vi "Create and Format PNG Image Link.vi"(8 "Error In":errorcluster, 11 "Image Name Cluster":T1) -> (0 "Error Out":errorcluster, 3 "Image Link":string)   [LabVIEW 2017]
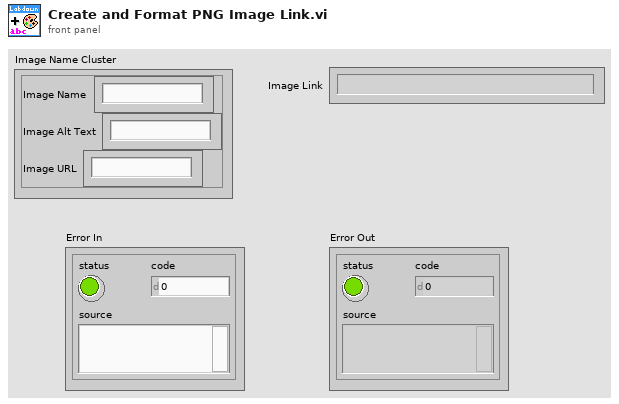
[diagram p1: front panel]
types:
  T1 = cluster{"Image Name":string, "Image Alt Text":string, "Image URL":string}
  T2 = enum16{"Header 1", "Header 2", "Header 3", "Header 4", "Header 5", "Header 6"}
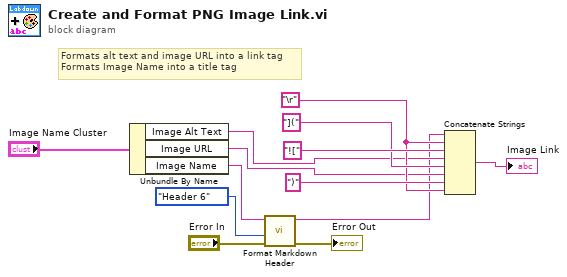
[diagram p0: block diagram]
diagram:
  w8 = "\r"
  # "Formats alt text and image URL into a link tag\nFormats Image Name into a title tag"
  n1 = Unbundle By Name("Image Name Cluster") -> ("Image Alt Text"=w4:string, "Image URL"=w2:string, "Image Name"=w3:string)
  n2 = call "Format Markdown Header.vi"("Error In"="Error In", "Header Size"=T2."Header 6", "Unformatted Heading Input"=w3) -> ("Error Out"=→"Error Out":errorcluster, "Formatted Header Output"=w1:string)  [unwired: 7 in]
  n3 = Concatenate Strings(w1, w8, "![", w4, "](", w2, ")", w8) -> (→"Image Link":string)
